vi "writeTestParametersFile.vi"(8 "error in (no error)":errorcluster, 11 "Logger in":refnum<class "Logger.lvclass">) -> (0 "error out":errorcluster, 3 "Logger out":refnum<class "Logger.lvclass">)   [LabVIEW 2013, in "Logger.lvclass"]
uses:
  Logger.lvclass
  Logger.lvclass/Logger.ctl
  <vilib>/Utility/file.llb/Write To Spreadsheet File (string).vi
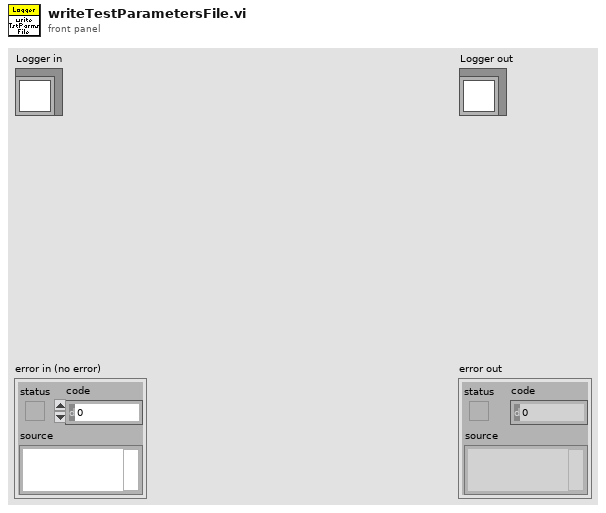
[diagram p1: front panel]
types:
  T1 = typedef "Test Parameters.ctl" = cluster{"Number of cycles for complete test":u32, "Cycle profile":T2, "Log Directory":path, "Max records per file":u32, "Comment":string}
  T2 = typedef "CycleProfileConfig.ctl" = cluster{"Force Setpoint":dbl[unit][], "Pause After":dbl[unit][]}
  T3 = typedef "System Controller.ctl" = cluster{"PID Gains":T4, "Force Error In Range Limit":dbl[unit]}
  T4 = typedef "PIDGains.ctl" = cluster{"Proportional Gain (Kc)":dbl, "Integral Time (Ti, min)":dbl, "Derivative Time (Td, min)":dbl}
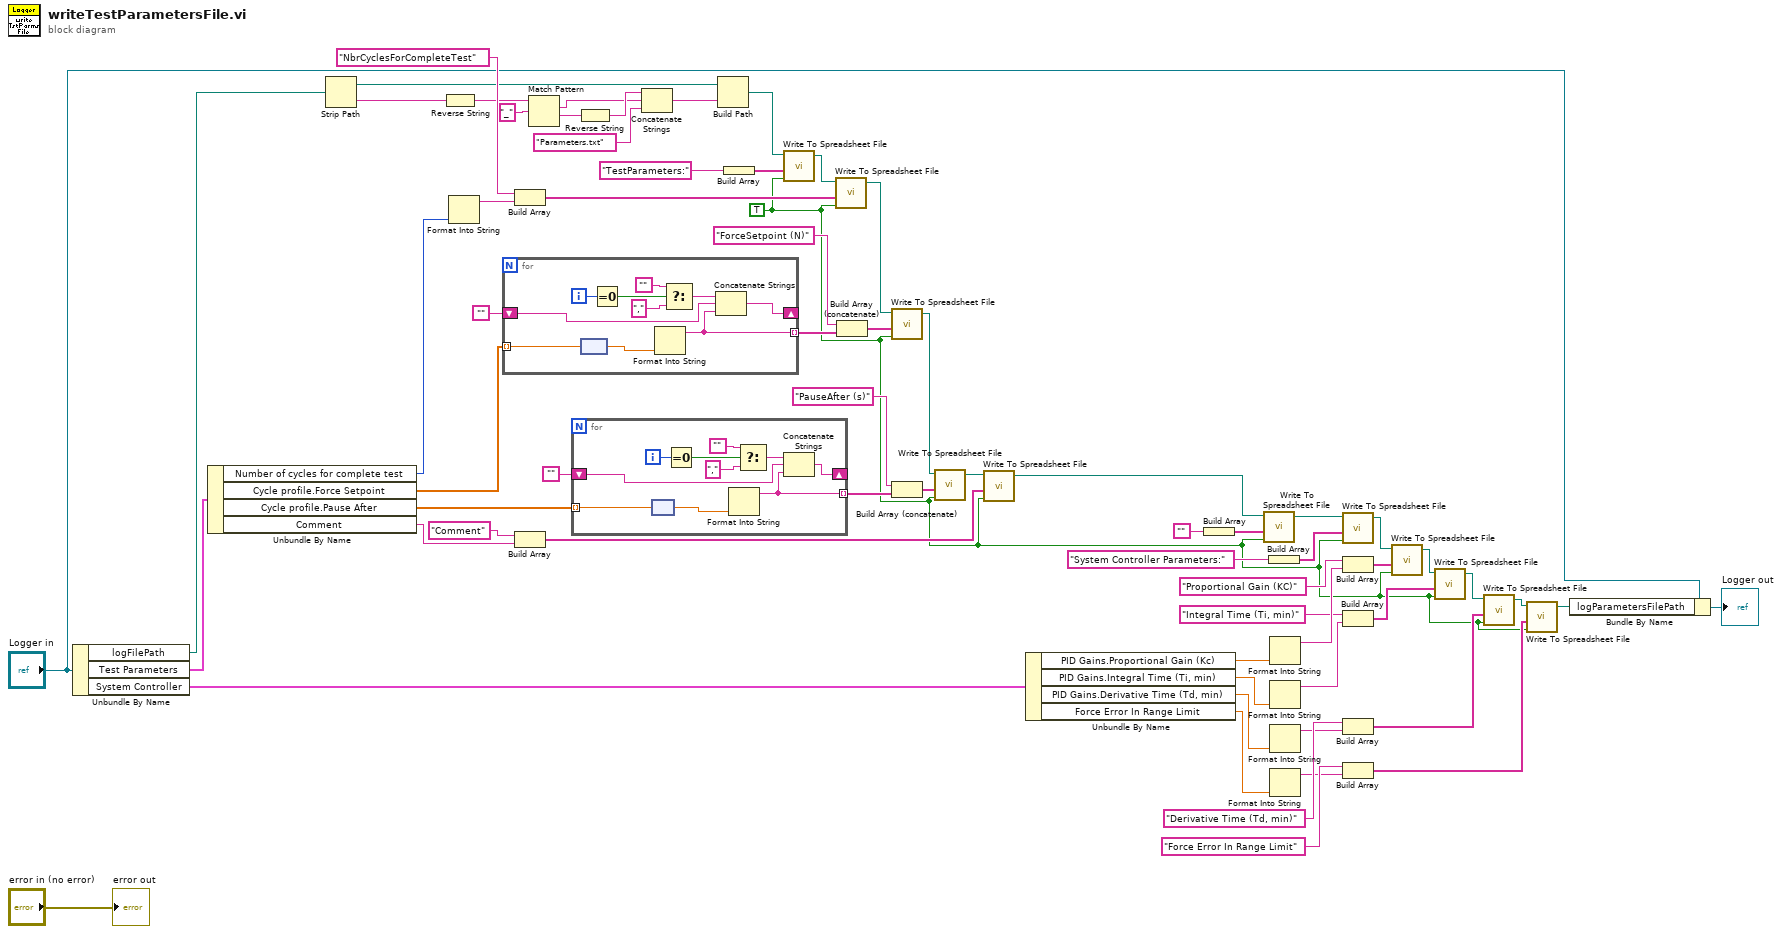
[diagram p0: block diagram]
diagram:
  w1 = TRUE ("append to file? (new file:F)")
  n1 = Unbundle By Name("Logger in") -> ("logFilePath"=w8:path, "Test Parameters"=w66:T1, "System Controller"=w37:T3)
  n2 = Unbundle By Name(w66) -> ("Number of cycles for complete test"=w65:u32, "Cycle profile.Force Setpoint"=w61:dbl[unit][], "Cycle profile.Pause After"=w57:dbl[unit][], "Comment"=w53:string)
  n3 = Strip Path(path=w8) -> (stripped path=w4:path, name=w13:string)
  n4 = Reverse String(1:w13) -> (0:w12:string)
  n5 = Format Into String(w65) -> (resulting string=w64:string)  [unwired: 3 in, 1 out]
  n6 = for {
    tunnel: w61 -> [w69] mode=indexing
    shift-right: [w77] -> _
    shift-left: "" -> [w76]
    tunnel: [w70] -> w47 mode=indexing
    i -> [w75]
    n7 = node(w69) -> (w68:dbl)
    n8 = Equal To 0?(x=w75) -> (x = 0?=w74:bool)
    n9 = Format Into String(w68) -> (resulting string=w70:string)  [unwired: 3 in, 1 out]
    n10 = Select(t="", s=w74, f=",") -> (s? t:f=w71:string)
    n11 = Concatenate Strings(w71, w76, w70) -> (w77:string)
  }
  n12 = Build Array("NbrCyclesForCompleteTest" ("element"), w64) -> (w63:string[])
  n13 = Build Array("Comment" ("element"), w53) -> (w52:string[])
  n14 = Match Pattern(string=w12, regular expression="_") -> (match substring=w2:string, after substring=w3:string)  [unwired: 1 in, 2 out]
  n15 = for {
    tunnel: w57 -> [w79] mode=indexing
    shift-right: [w87] -> _
    shift-left: "" -> [w86]
    tunnel: [w80] -> w46 mode=indexing
    i -> [w85]
    n16 = node(w79) -> (w78:dbl)
    n17 = Equal To 0?(x=w85) -> (x = 0?=w84:bool)
    n18 = Format Into String(w78) -> (resulting string=w80:string)  [unwired: 3 in, 1 out]
    n19 = Select(t="", s=w84, f=",") -> (s? t:f=w81:string)
    n20 = Concatenate Strings(w81, w86, w80) -> (w87:string)
  }
  n21 = Reverse String(1:w3) -> (0:w10:string)
  n22 = Concatenate Strings(w10, w2, "Parameters.txt" ("string")) -> (w7:string)
  n23 = Build Path(base path=w4, name or relative path=w7) -> (appended path=w6:path)
  n24 = Build Array("TestParameters:") -> (w41:string[])
  n25 = call-poly <vilib>:"Write To Spreadsheet File.vi"("append to file? (new file:F)"=w1, "1D data"=w41, "file path (dialog if empty)"=w6) -> ("new file path (Not A Path if cancelled)"=w43:path)  [unwired: 5 in]
  n26 = call-poly <vilib>:"Write To Spreadsheet File.vi"("append to file? (new file:F)"=w1, "1D data"=w63, "file path (dialog if empty)"=w43) -> ("new file path (Not A Path if cancelled)"=w62:path)  [unwired: 5 in]
  n27 = Build Array (concatenate)("ForceSetpoint (N)" ("element"), w47) -> (w59:string[])
  n28 = call-poly <vilib>:"Write To Spreadsheet File.vi"("append to file? (new file:F)"=w1, "1D data"=w59, "file path (dialog if empty)"=w62) -> ("new file path (Not A Path if cancelled)"=w58:path)  [unwired: 5 in]
  n29 = Build Array (concatenate)("PauseAfter (s)" ("element"), w46) -> (w55:string[])
  n30 = call-poly <vilib>:"Write To Spreadsheet File.vi"("append to file? (new file:F)"=w1, "1D data"=w55, "file path (dialog if empty)"=w58) -> ("new file path (Not A Path if cancelled)"=w54:path)  [unwired: 5 in]
  n31 = call-poly <vilib>:"Write To Spreadsheet File.vi"("append to file? (new file:F)"=w1, "1D data"=w52, "file path (dialog if empty)"=w54) -> ("new file path (Not A Path if cancelled)"=w40:path)  [unwired: 5 in]
  n32 = Unbundle By Name(w37) -> ("PID Gains.Proportional Gain (Kc)"=w34:dbl, "PID Gains.Integral Time (Ti, min)"=w28:dbl, "PID Gains.Derivative Time (Td, min)"=w22:dbl, "Force Error In Range Limit"=w20:dbl[unit])
  n33 = Build Array("") -> (w44:string[])
  n34 = call-poly <vilib>:"Write To Spreadsheet File.vi"("append to file? (new file:F)"=w1, "1D data"=w44, "file path (dialog if empty)"=w40) -> ("new file path (Not A Path if cancelled)"=w18:path)  [unwired: 5 in]
  n35 = Build Array("System Controller Parameters:" ("element")) -> (w35:string[])
  n36 = Format Into String(w34) -> (resulting string=w32:string)  [unwired: 3 in, 1 out]
  n37 = Format Into String(w28) -> (resulting string=w27:string)  [unwired: 3 in, 1 out]
  n38 = Format Into String(w22) -> (resulting string=w21:string)  [unwired: 3 in, 1 out]
  n39 = Format Into String(w20) -> (resulting string=w19:string)  [unwired: 3 in, 1 out]
  n40 = call-poly <vilib>:"Write To Spreadsheet File.vi"("append to file? (new file:F)"=w1, "1D data"=w35, "file path (dialog if empty)"=w18) -> ("new file path (Not A Path if cancelled)"=w17:path)  [unwired: 5 in]
  n41 = Build Array("Proportional Gain (KC)" ("element"), w32) -> (w31:string[])
  n42 = Build Array("Integral Time (Ti, min)" ("element"), w27) -> (w29:string[])
  n43 = Build Array("Derivative Time (Td, min)" ("element"), w21) -> (w24:string[])
  n44 = Build Array("Force Error In Range Limit" ("element"), w19) -> (w23:string[])
  n45 = call-poly <vilib>:"Write To Spreadsheet File.vi"("append to file? (new file:F)"=w1, "1D data"=w31, "file path (dialog if empty)"=w17) -> ("new file path (Not A Path if cancelled)"=w16:path)  [unwired: 5 in]
  n46 = call-poly <vilib>:"Write To Spreadsheet File.vi"("append to file? (new file:F)"=w1, "1D data"=w29, "file path (dialog if empty)"=w16) -> ("new file path (Not A Path if cancelled)"=w15:path)  [unwired: 5 in]
  n47 = call-poly <vilib>:"Write To Spreadsheet File.vi"("append to file? (new file:F)"=w1, "1D data"=w24, "file path (dialog if empty)"=w15) -> ("new file path (Not A Path if cancelled)"=w14:path)  [unwired: 5 in]
  n48 = call-poly <vilib>:"Write To Spreadsheet File.vi"("append to file? (new file:F)"=w1, "1D data"=w23, "file path (dialog if empty)"=w14) -> ("new file path (Not A Path if cancelled)"=w5:path)  [unwired: 5 in]
  n49 = Bundle By Name(cluster="Logger in", "logParametersFilePath"=w5) -> (→"Logger out":refnum<class "Logger.lvclass">)
  "error out" <- "error in (no error)"
